vi "Choix Caméra 1P.vi"(9 "Detecté caméra D":bool, 11 "Detecté caméra G":bool) -> (0 "Choix":u16, 1 "Detecté caméra D":bool, 2 "Detecté caméra G et D":bool, 3 "Detecté caméra G":bool)   [LabVIEW 2013]
panel:
  # "Détection et allumage de LED"
  # "Choix :\n0 = pas de pokaenmon détecté\n1 = pokaenmon détecté par la caméra de gauche seulement\n2 = pokaenmon détecté par les deux caméras\n3 = pokaenmon détecté par la caméra de droite seulement"
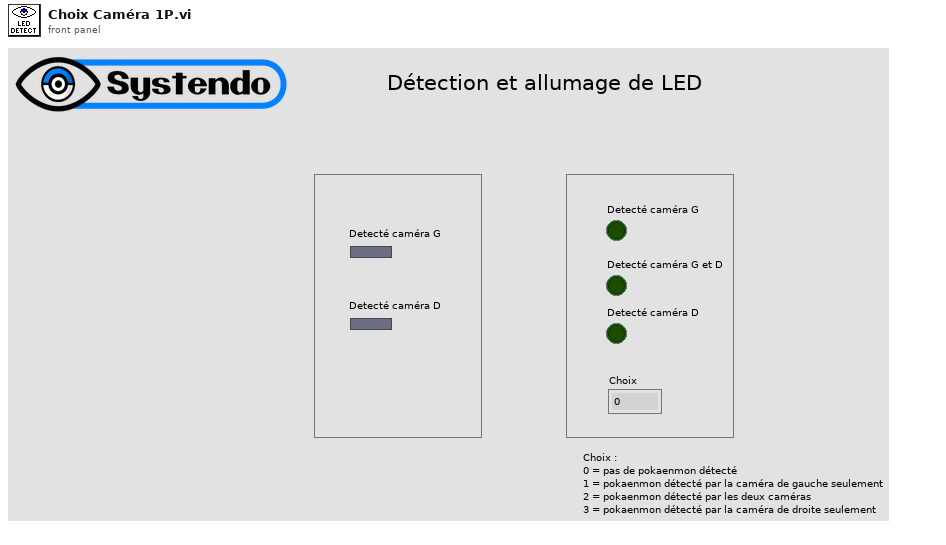
[diagram p1: front panel]
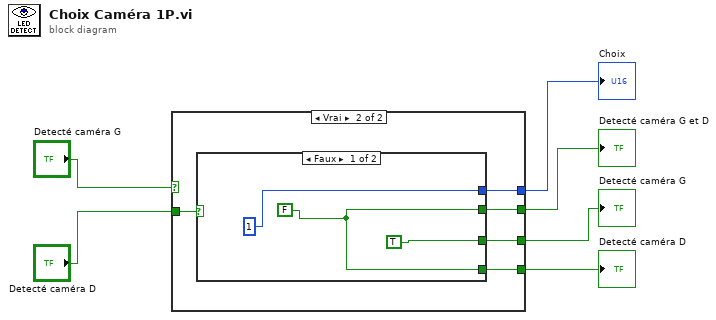
[diagram p0: block diagram]
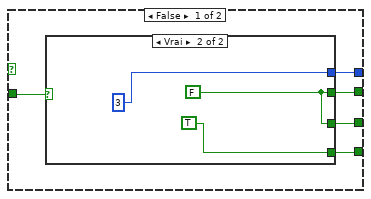
[diagram p2: hidden frame]
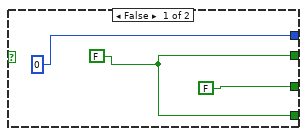
[diagram p3: hidden frame]
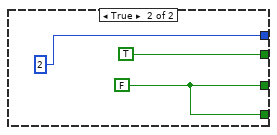
[diagram p4: hidden frame]
diagram:
  n1 = case shown="Vrai" "Detecté caméra G" {
    tunnel: [w8 w22] -> w5
    tunnel: [w9 w21] -> w4
    tunnel: [w10 w20] -> w3
    tunnel: "Detecté caméra D" -> [w11 w19]
    tunnel: [w7 w18] -> w1
    frame False {
      n2 = case shown="Vrai" w11 {
        tunnel: [w13 w16] -> w8
        tunnel: [FALSE w16] -> w9
        tunnel: [w13 TRUE] -> w10
        tunnel: [0 3] -> w7
        frame False {
          w13 = FALSE
        }
        frame True {
          w16 = FALSE
        }
      }
    }
    frame True {
      n3 = case shown="Faux" w19 {
        tunnel: [w24 TRUE] -> w22
        tunnel: [TRUE w27] -> w21
        tunnel: [w24 w27] -> w20
        tunnel: [1 2] -> w18
        frame False {
          w24 = FALSE
        }
        frame True {
          w27 = FALSE
        }
      }
    }
  }
  "Detecté caméra G" <- w4
  "Detecté caméra D" <- w3
  "Detecté caméra G et D" <- w5
  "Choix" <- w1
